vi "Variable globale Ctrl State SMC100.vi"() -> ()   [LabVIEW 2024]
panel:
  in  "controllerState":string
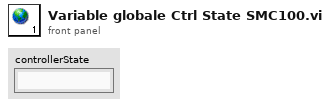
[diagram p1: front panel]
diagram:
